vi "Periodic Tasks.vi"(8 "error in":errorcluster) -> ()   [LabVIEW 2013]
doc: "This VI runs in parallel to other tasks. It can contain as many user-defined periodic loops as you need. These can carry out PID or other sorts of timed response."
uses:
  <vilib>/Rock Robotics/SystemInterfaces/Utilities/FPGA_UtilitiesLED Source.ctl
  <vilib>/Rock Robotics/SystemInterfaces/Utilities/FPGA_UtilitiesLED State.ctl
  Robot Global Data.vi
  <vilib>/Rock Robotics/WPI/Joystick/WPI_JoystickGetSetRefNum.vi
  <vilib>/Rock Robotics/WPI/RobotDrive/WPI_RobotDriveGetSetRefNum.vi
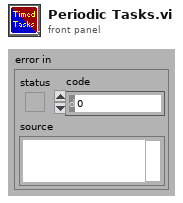
[diagram p1: front panel]
types:
  T1 = typedef "WPI_MotorControlDeviceRef.ctl" = cluster{"DeviceStatus":errorcluster, "Type":enum16{"PWM", "CAN"}, "PWM":cluster{"Digital Module":T2, "PWM Channel":T3, "DeadBand":T4}, "CAN":cluster{"Device Number":u8, "Control Mode":T5, "Semaphore":T6, "Max Vout":dbl}, "Invert":bool, "TransformRef":T7, "InvTransformRef":T7}
  T2 = typedef "FPGA_TypedefDigitalModule.ctl" = enum16{"Digital Module 1", "Digital Module 2"}
  T3 = typedef "FPGA_DIOPWMChannel.ctl" = enum8{"PWM 1", "PWM 2", "PWM 3", "PWM 4", "PWM 5", "PWM 6", "PWM 7", "PWM 8", "PWM 9", "PWM 10", "Invalid"}
  T4 = typedef "WPI_PWMDeadband.ctl" = cluster{"Name":string, "maxPositivePwm":i32, "minPositivePwm":i32, "centerPwm":i32, "maxNegativePwm":i32, "minNegativePwm":i32, "angularRange":u16}
  T5 = typedef "WPI_CANJaguar_ControlMode.ctl" = enum8{"Percent VBus", "Current", "Speed", "Position", "Voltage"}
  T6 = typedef "Semaphore RefNum" = refnum<k1>
  T7 = typedef "WPI_PWMTransform_ConPane.ctl" = refnum<vi>
  T8 = typedef "WPI_JoystickDevRef.ctl" = cluster{"Device":T9}
  T9 = typedef "WPI_JoystickDeviceEnum.ctl" = enum16{"USB 1", "USB 2", "USB 3", "USB 4", "Kinect 1", "Kinect 2"}
  T10 = typedef "WPI_DigitalInputDevRef.ctl" = cluster{"DevStatus":errorcluster, "DIO Channel":T11, "Digital Module":T2}
  T11 = typedef "FPGA_DIOChannel.ctl" = enum8{"DIO 1", "DIO 2", "DIO 3", "DIO 4", "DIO 5", "DIO 6", "DIO 7", "DIO 8", "DIO 9", "DIO 10", "DIO 11", "DIO 12", "DIO 13", "DIO 14", "Invalid"}
  T12 = typedef "WPI_JoystickButtonState.ctl" = cluster{"Button 1":bool, "Button 2":bool, "Button 3":bool, "Button 4":bool, "Button 5":bool, "Button 6":bool, "Button 7":bool, "Button 8":bool, "Button 9":bool, "Button 10":bool, "Button 11":bool, "Button 12":bool}
  T13 = typedef "WPI_RobotDriveDevRef.ctl" = cluster{"DevStatus":errorcluster, "Motors[]":T1[], "Square Inputs":bool, "Max Output":dbl, "Isochronous":bool}
  T14 = cluster{"JoystickDevRef":T8, "RobotDriveDevRef":T13}
  T15 = typedef "FPGA_UtilitiesLED State.ctl" = enum16{"Off", "On", "Toggle"}
  T16 = typedef "FPGA_UtilitiesLED Source.ctl" = enum16{"User LED", "FPGA LED"}
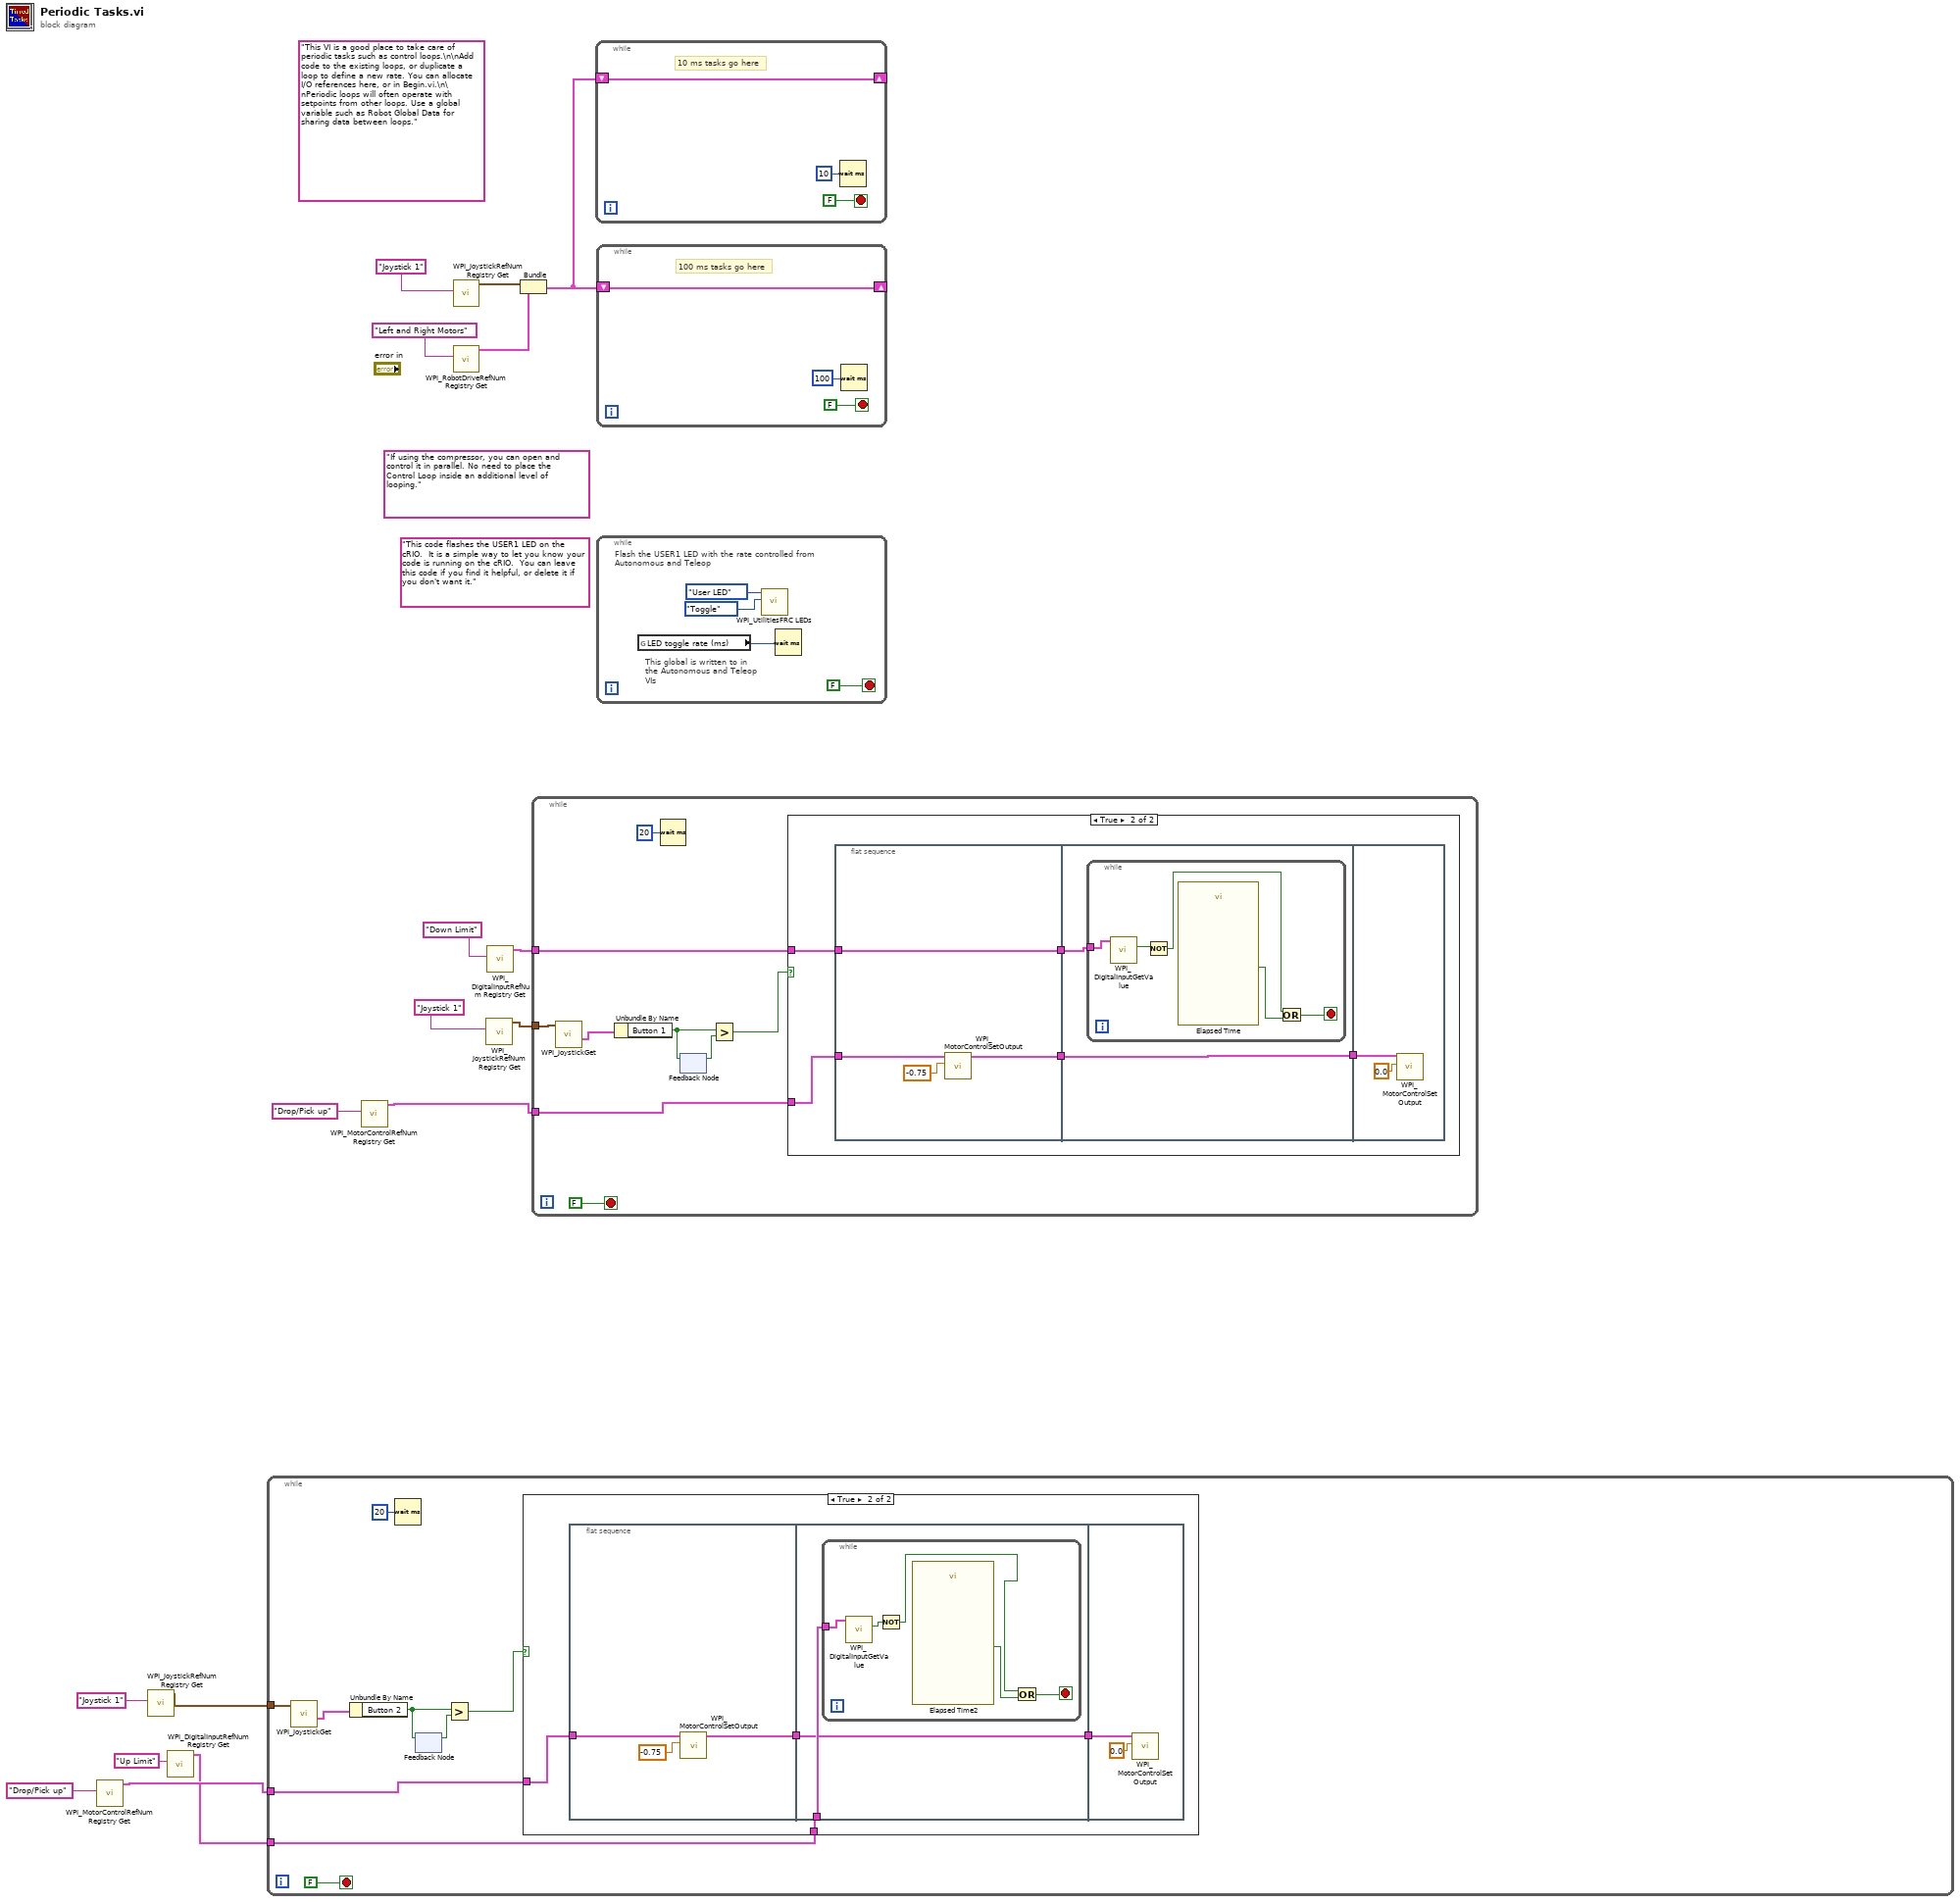
[diagram p0: block diagram]
diagram:
  (unwired) "If using the compressor, you can open and control it in parallel. No need to place the Control Loop inside an additional level of looping."
  (unwired) "This code flashes the USER1 LED on the cRIO.  It is a simple way to let you know your code is running on the cRIO.  You can leave this code if you find it helpful, or delete it if you don't want it."
  (unwired) "This VI is a good place to take care of periodic tasks such as control loops.\n\nAdd code to the existing loops, or duplicate a loop to define a new rate. You can allocate I/O references here, or in Begin.vi.\n\nPeriodic loops will often operate with setpoints from other loops. Use a global variable such as Robot Global Data for sharing data between loops."
  n1 = call <vilib>:"WPI_MotorControlRefNum Registry Get.vi"("refnum name"="Drop/Pick up") -> ("MotorControlDevRef"=w7:T1)  [unwired: 9 in, 1 out]
  n2 = call <vilib>:"WPI_JoystickRefNum Registry Get.vi"("refnum name"="Joystick 1") -> ("JoystickDevRef"=w8:T8)  [unwired: 9 in, 1 out]
  n3 = call <vilib>:"WPI_DigitalInputRefNum Registry Get.vi"("refnum name"="Up Limit") -> ("DigitalInputDevRef"=w4:T10)  [unwired: 9 in, 1 out]
  n4 = while {
    tunnel: w8 -> [w25]
    tunnel: w7 -> [w20]
    tunnel: w4 -> [w18]
    stop <- FALSE stop-if-true
    n5 = call <vilib>:"WPI_JoystickGet.vi"("JoystickDevRef"=w25) -> ("Buttons"=w24:T12)  [unwired: 4 in, 2 out]
    n6 = Unbundle By Name(w24) -> ("Button 2"=w22:bool)
    n7 = Wait (ms)(milliseconds to wait=u32 20) -> ()  [unwired: 1 out]
    n8 = feedback-in #1(w22) -> ()
    n9 = feedback #1() -> (w23:bool)  [unwired: 1 in]
    n10 = Greater?(x=w22, y=w23) -> (0:w21:bool)
    n11 = case shown="True" w21 {
      tunnel: w20 -> [_ w30]
      tunnel: w18 -> [_ w27]
      frame False {
      }
      frame True {
        n12 = flat-sequence {
          tunnel: w30 -> [w33]
          tunnel: [w32] -> w29
          tunnel: w29 -> [w34]
          tunnel: [w34] -> w28
          tunnel: w27 -> [w35]
          tunnel: w28 -> [w42]
          frame #0 {
            n13 = call <vilib>:"WPI_MotorControlSetOutput.vi"("Output"=-0.75, "MotorControlDevRef"=w33) -> ("MotorControlDevRef"=w32:T1)  [unwired: 7 in, 2 out]
          }
          frame #1 {
            n14 = while {
              tunnel: w35 -> [w40]
              stop <- w38 stop-if-true
              n15 = call <vilib>:"WPI_DigitalInputGetValue.vi"("DigitalInputDevRef"=w40) -> ("Value"=w37:bool)  [unwired: 8 in, 2 out]
              n16 = Not(x=w37) -> (.not. x?=w36:bool)
              n17 = call "Elapsed Time2"() -> ("Time has Elapsed"=w39:bool)  [unwired: 12 in, 7 out]
              n18 = Or(x=w36, y=w39) -> (x .or. y?=w38:bool)
            }
          }
          frame #2 {
            n19 = call <vilib>:"WPI_MotorControlSetOutput.vi"("Output"=0.0, "MotorControlDevRef"=w42) -> ()  [unwired: 7 in, 3 out]
          }
        }
      }
    }
  }
  n20 = call <vilib>:"WPI_MotorControlRefNum Registry Get.vi"("refnum name"="Drop/Pick up") -> ("MotorControlDevRef"=w11:T1)  [unwired: 9 in, 1 out]
  n21 = call <vilib>:"WPI_JoystickRefNum Registry Get.vi"("refnum name"="Joystick 1") -> ("JoystickDevRef"=w15:T8)  [unwired: 1 in, 9 out]
  n22 = call <vilib>:"WPI_RobotDriveRefNum Registry Get.vi"("refnum name"="Left and Right Motors") -> ("RobotDriveDevRef"=w14:T13)  [unwired: 1 in, 9 out]
  n23 = call <vilib>:"WPI_JoystickRefNum Registry Get.vi"("refnum name"="Joystick 1") -> ("JoystickDevRef"=w3:T8)  [unwired: 9 in, 1 out]
  n24 = call <vilib>:"WPI_DigitalInputRefNum Registry Get.vi"("refnum name"="Down Limit") -> ("DigitalInputDevRef"=w1:T10)  [unwired: 9 in, 1 out]
  n25 = Bundle("JoystickDevRef"=w15, "RobotDriveDevRef"=w14) -> (w13:T14)  [unwired: 1 out]
  n26 = while {
    tunnel: w11 -> [w46]
    tunnel: w3 -> [w44]
    tunnel: w1 -> [w43]
    stop <- FALSE stop-if-true
    n27 = call <vilib>:"WPI_JoystickGet.vi"("JoystickDevRef"=w44) -> ("Buttons"=w50:T12)  [unwired: 4 in, 2 out]
    n28 = Unbundle By Name(w50) -> ("Button 1"=w48:bool)
    n29 = Wait (ms)(milliseconds to wait=u32 20) -> ()  [unwired: 1 out]
    n30 = feedback-in #2(w48) -> ()
    n31 = feedback #2() -> (w49:bool)  [unwired: 1 in]
    n32 = Greater?(x=w48, y=w49) -> (0:w47:bool)
    n33 = case shown="True" w47 {
      tunnel: w46 -> [_ w56]
      tunnel: w43 -> [_ w52]
      frame False {
      }
      frame True {
        n34 = flat-sequence {
          tunnel: w56 -> [w60]
          tunnel: [w59] -> w55
          tunnel: [w57] -> w53
          tunnel: w52 -> [w57]
          tunnel: w55 -> [w62]
          tunnel: [w62] -> w54
          tunnel: w53 -> [w61]
          tunnel: w54 -> [w69]
          frame #0 {
            n35 = call <vilib>:"WPI_MotorControlSetOutput.vi"("Output"=-0.75, "MotorControlDevRef"=w60) -> ("MotorControlDevRef"=w59:T1)  [unwired: 7 in, 2 out]
          }
          frame #1 {
            n36 = while {
              tunnel: w61 -> [w67]
              stop <- w65 stop-if-true
              n37 = call <vilib>:"WPI_DigitalInputGetValue.vi"("DigitalInputDevRef"=w67) -> ("Value"=w64:bool)  [unwired: 8 in, 2 out]
              n38 = Not(x=w64) -> (.not. x?=w63:bool)
              n39 = call "Elapsed Time"() -> ("Time has Elapsed"=w66:bool)  [unwired: 12 in, 7 out]
              n40 = Or(x=w63, y=w66) -> (x .or. y?=w65:bool)
            }
          }
          frame #2 {
            n41 = call <vilib>:"WPI_MotorControlSetOutput.vi"("Output"=0.0, "MotorControlDevRef"=w69) -> ()  [unwired: 7 in, 3 out]
          }
        }
      }
    }
  }
  n42 = while {
    shift-right: [w70] -> _
    shift-left: w13 -> [w70]
    stop <- FALSE stop-if-true
    # "10 ms tasks go here"
    n43 = Wait (ms)(milliseconds to wait=u32 10) -> ()  [unwired: 1 out]
  }
  n44 = while {
    shift-right: [w73] -> _
    shift-left: w13 -> [w73]
    stop <- FALSE stop-if-true
    # "100 ms tasks go here"
    n45 = Wait (ms)(milliseconds to wait=u32 100) -> ()  [unwired: 1 out]
  }
  n46 = while {
    stop <- FALSE stop-if-true
    # "This global is written to in the Autonomous and Teleop VIs"
    # "Flash the USER1 LED with the rate controlled from Autonomous and Teleop"
    n47 = global read "Robot Global Data.vi" "LED toggle rate (ms)"() -> (w76:u32)
    n48 = call <vilib>:"WPI_UtilitiesFRC LEDs.vi"("State"=FPGA_UtilitiesLED_State."Toggle", "LED Type"=FPGA_UtilitiesLED_Source."User LED") -> ()  [unwired: 1 in, 9 out]
    n49 = Wait (ms)(milliseconds to wait=w76) -> ()  [unwired: 1 out]
  }
